vi "Create Logger Prep.vi"(7 "Timestamp":string, 8 "error in (no error)":errorcluster, 11 "Historian Logger in":refnum<class "Historian Logger.lvclass">) -> (0 "error out":errorcluster, 2 "Logger Info":T1, 3 "Historian Logger out":refnum<class "Historian Logger.lvclass">)   [LabVIEW 2020, in "VolatusHistorian.lvlib" / "Historian Logger.lvclass"]
uses:
  Historian Logger.lvclass
  VolatusData/Prepare Log.ctl
  Historian Logger.lvclass/Historian Logger.ctl
  VolatusData/VolatusData.lvlib
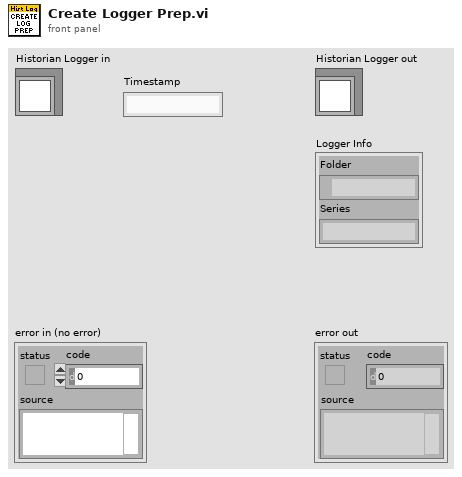
[diagram p1: front panel]
types:
  T1 = typedef "VolatusData.lvlib/Prepare Log.ctl" = cluster{"Folder":path, "Series":string}
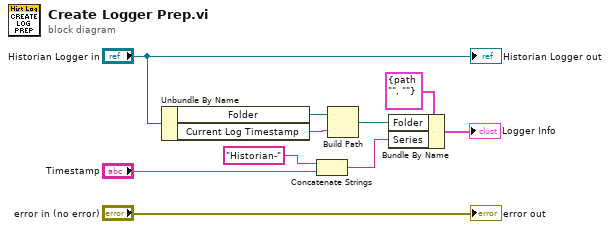
[diagram p0: block diagram]
diagram:
  n1 = Unbundle By Name("Historian Logger in") -> ("Folder"=w7:path, "Current Log Timestamp"=w6:string)
  n2 = Concatenate Strings("Historian-" ("Series"), "Timestamp") -> (w2:string)
  n3 = Build Path(base path=w7, name or relative path=w6) -> (appended path=w5:path)
  n4 = Bundle By Name(cluster=T1 {"Folder"=path "", "Series"=""} ("Prepare Log"), "Folder"=w5, "Series"=w2) -> (→"Logger Info":T1)
  "error out" <- "error in (no error)"
  "Historian Logger out" <- "Historian Logger in"
